vi "Test_Create.vi"() -> (0 "error out":errorcluster, 3 "Maui.Config out":refnum<class "Maui.Config.lvclass">)   [LabVIEW 2020, in "Test_Maui.Config.lvclass"]
uses:
  Test_Maui.Config.lvclass
  lvsrc/Maui.Config/Maui.Config.lvclass
  <vilib>/Utility/sysdir.llb/System Directory Type.ctl
  lvsrc/SMO.UI.MAUI.lvclass
  <vilib>/addons/_JKI Toolkits/Caraya/classes/Assert/Assert True.vi
  <vilib>/addons/_JKI Toolkits/Caraya/classes/Assert/Assert Equal Value and Type_Variant.vi
  <vilib>/addons/_JKI Toolkits/Caraya/classes/Assert/Assert Equal Value_Variant.vi
  <vilib>/addons/_JKI Toolkits/Caraya/classes/Test/Test.lvclass
  <vilib>/addons/_JKI Toolkits/Caraya/classes/Assert/Assert.lvclass
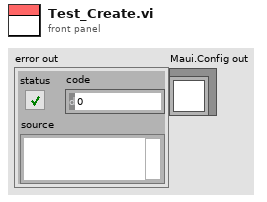
[diagram p1: front panel]
types:
  T1 = typedef "System Directory Type.ctl" = i32
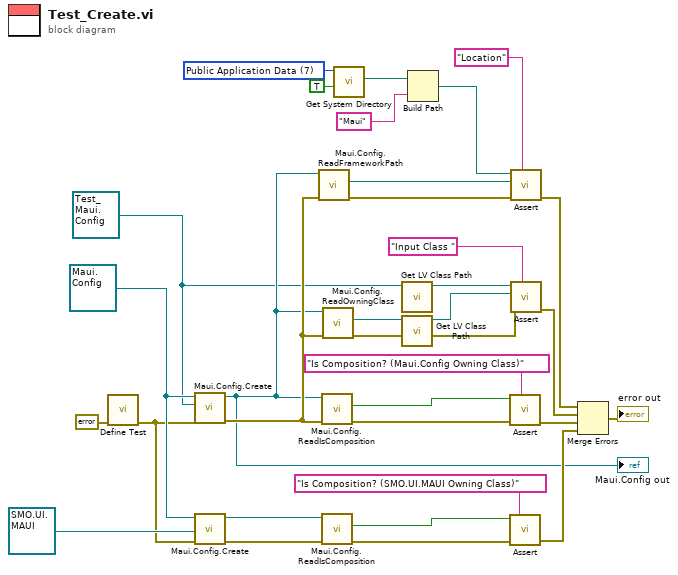
[diagram p0: block diagram]
diagram:
  w26 = T1 7 items=["User Home"=0, "User Desktop"=1, "User Documents"=2, "User Application Data"=3, "User Preferences"=4, "User Temporary"=5, "Public Documents"=6, "Public Application Data"=7, "Public Preferences"=8, "Public Cache"=13, "System Core Libraries"=9, "System Installed Libraries"=10, "Application Files"=11, "Boot Volume Root"=12] ("system directory type")
  w3 = refnum<class "Test_Maui.Config.lvclass"> refnum ("Test_Maui.Config.lvclass")
  w10 = refnum<class "Maui.Config.lvclass"> refnum ("Maui.Config in")
  n1 = call <vilib>:"Define Test.vi"("error in (no error)"=errorcluster {"status"=FALSE, "code"=0, "source"=""}) -> ("error out"=w2:errorcluster)  [unwired: 10 in]
  n2 = call "Maui.Config.Create.vi"("error in (no error)"=w2, "Owning Class"=w3, "Maui.Config in"=w10) -> ("error out"=w12:errorcluster, "Maui.Config out"=w4:refnum<class "Maui.Config.lvclass">)  [unwired: 7 in]
  "Maui.Config out" <- w4
  n3 = call "Maui.Config.Create.vi"("error in (no error)"=w2, "Owning Class"=refnum<class "SMO.UI.MAUI.lvclass"> refnum ("SMO.UI.MAUI.lvclass"), "Maui.Config in"=w10) -> ("error out"=w13:errorcluster, "Maui.Config out"=w16:refnum<class "Maui.Config.lvclass">)  [unwired: 7 in]
  n4 = call "Maui.Config.ReadFrameworkPath.vi"("error in (no error)"=w12, "Maui.Config in"=w4) -> ("error out"=w21:errorcluster, "Framework Path"=w20:path)  [unwired: 7 in, 1 out]
  n5 = call "Maui.Config.ReadIsComposition.vi"("error in (no error)"=w12, "Maui.Config in"=w4) -> ("error out"=w29:errorcluster, "Composition"=w30:bool)  [unwired: 7 in, 1 out]
  n6 = call "Maui.Config.ReadIsComposition.vi"("error in (no error)"=w13, "Maui.Config in"=w16) -> ("error out"=w15:errorcluster, "Composition"=w14:bool)  [unwired: 7 in, 1 out]
  n7 = call "Maui.Config.ReadOwningClass.vi"("error in (no error)"=w12, "Maui.Config in"=w4) -> ("error out"=w1:errorcluster, "Owning Class"=w8:refnum<class>)  [unwired: 7 in, 1 out]
  n8 = call <vilib>:"Get System Directory.vi"("create directory if not found? (F)"=TRUE, "system directory type"=w26) -> ("system directory"=w25:path)  [unwired: 9 in]
  n9 = call <vilib>:"Get LV Class Path.vi"("object"=w3) -> ("class path"=w6:path)  [unwired: 9 in, 1 out]
  n10 = call <vilib>:"Get LV Class Path.vi"("object"=w8) -> ("class path"=w7:path)  [unwired: 9 in, 1 out]
  n11 = Build Path(base path=w25, name or relative path="Maui") -> (appended path=w19:path)
  n12 = call-poly <vilib>:"Assert.vi"("Label"="Is Composition? (Maui.Config Owning Class)" ("Label (VI Title)"), "error in (no error)"=w29, "True?"=w30) -> ("error out"=w32:errorcluster)  [unwired: 8 in]
  n13 = call-poly <vilib>:"Assert.vi"("Label"="Is Composition? (SMO.UI.MAUI Owning Class)" ("Label (VI Title)"), "error in (no error)"=w15, "True?"=w14) -> ("error out"=w5:errorcluster)  [unwired: 8 in]
  n14 = call-poly <vilib>:"Assert.vi"("Label"="Location", "error in (no error)"=w21, "Y"=w20, "X"=w19) -> ("error out"=w18:errorcluster)  [unwired: 7 in]
  n15 = call-poly <vilib>:"Assert.vi"("Label"="Input Class ", "error in (no error)"=w1, "Y"=w7, "X"=w6) -> ("error out"=w27:errorcluster)  [unwired: 7 in]
  n16 = Merge Errors(w18, w27, w32, w5) -> (→"error out":errorcluster)
